vi "GP354 Ion Guage.vi"(0 "CloseVi?":bool) -> ()   [LabVIEW 2011]
panel:
  in  "Close Button":bool
  out "Output Byte 0":u8
  in  "Input Byte 2":u8
  in  "Input Byte 1":u8
  in  "Input Byte 0":u8
  in  "High Emission":bool
  in  "Ion Gauge":bool
  in  "Medium Emission":bool
  in  "Enable Filament 2":bool
  in  "Enable Filament 1":bool
  in  "Degas":bool
  out "Warnings":bool
  out "Alarms":bool
  out "Pressure":dbl
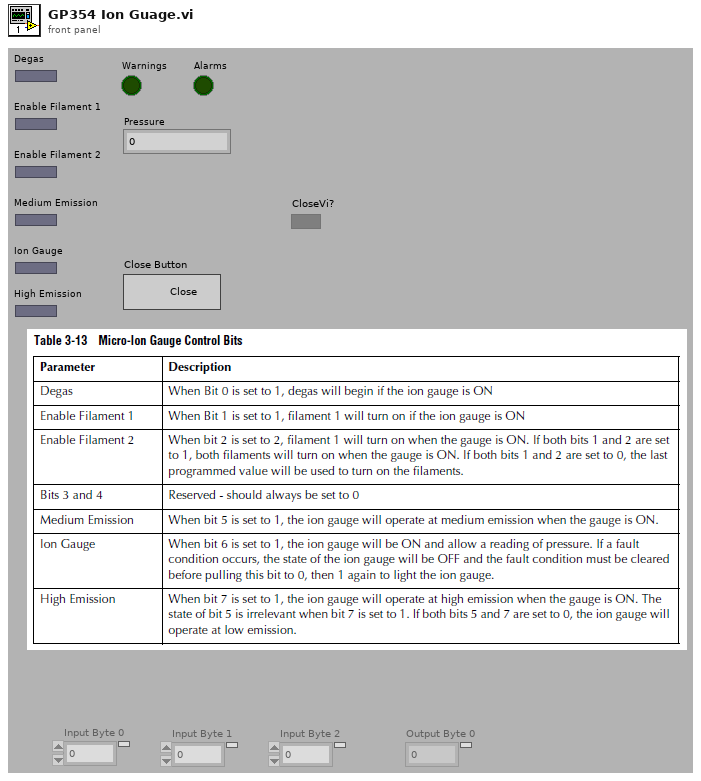
[diagram p1: front panel]
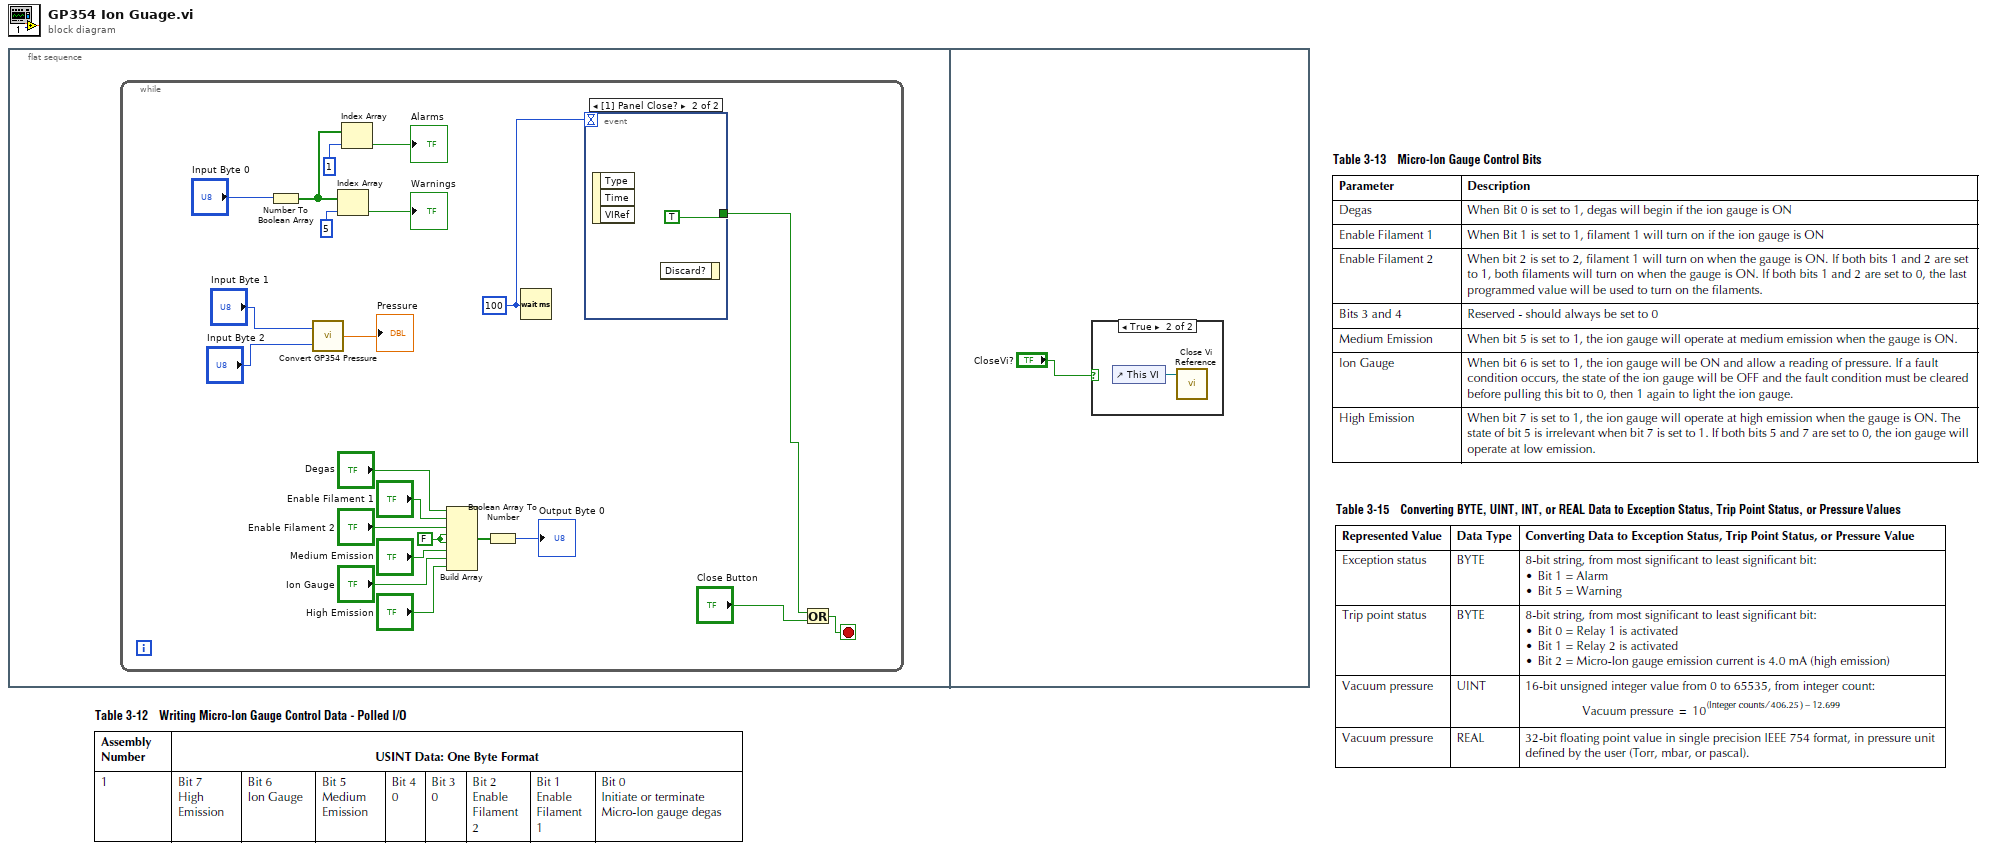
[diagram p0: block diagram]
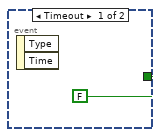
[diagram p2: hidden frame]
diagram:
  n1 = flat-sequence {
    frame #0 {
      n2 = while {
        stop <- w12 stop-if-true
        w2 = FALSE
        w13 = 100
        n3 = Number To Boolean Array(number="Input Byte 0") -> (Boolean array=w22:bool[])
        n4 = call "Convert GP354 Pressure.vi"("Input Byte 2"="Input Byte 2", "Input Byte 1"="Input Byte 1") -> ("Pressure"=→"Pressure":dbl)
        n5 = Index Array(array=w22, index=i8 5) -> (element=→"Warnings":bool)
        n6 = Index Array(array=w22, index=i8 1) -> (element=→"Alarms":bool)
        n7 = Build Array("Degas", "Enable Filament 1", "Enable Filament 2", w2, w2, "Medium Emission", "Ion Gauge", "High Emission") -> (w5:bool[])
        n8 = Boolean Array To Number(Boolean array=w5) -> (number=→"Output Byte 0":u8)
        n9 = Wait (ms)(milliseconds to wait=w13) -> ()  [unwired: 1 out]
        n10 = event shown="[1] Panel Close?" {
          selector: _ -> [_ _]
          dyn-events: _ -> [_ _]
          timeout: w13 -> [_ _]
          tunnel: [FALSE ("y") TRUE ("y")] -> w10
          event Timeout {
            n11 = event-data() -> ()  [unwired: 1 in, 2 out]
          }
          event Panel Close? {
            n12 = event-data() -> ()  [unwired: 1 in, 3 out]
            n13 = event-data() -> ()  [unwired: 2 in, 1 out]
          }
        }
        n14 = Or(x=w10, y="Close Button") -> (x .or. y?=w12:bool)
      }
    }
    frame #1 {
      n15 = case shown="True" "CloseVi?" {
        frame False {
        }
        frame True {
          n16 = control-ref of="This VI"() -> (w26:refnum<vi>)
          n17 = call "Close Vi Reference.vi"("reference"=w26) -> ()  [unwired: 9 in, 2 out]
        }
      }
    }
  }
